vi "__Local List Menu Upload Handler.vi"(7 "FileManager Data":T1, 8 "error in (no error)":errorcluster) -> (0 "error out":errorcluster)   [LabVIEW 2011]
doc: "Handles the upload operation on the Local list."
uses:
  __File manager Data type.ctl
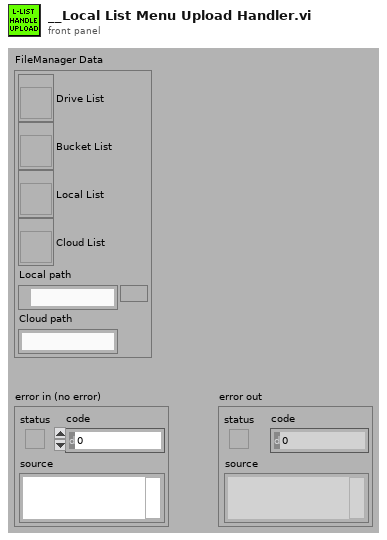
[diagram p1: front panel]
types:
  T1 = typedef "__File manager Data type.ctl" = cluster{"Drive List":refnum<vi>, "Bucket List":refnum<vi>, "Local List":refnum<vi>, "Cloud List":refnum<vi>, "Local path":path, "Cloud path":string}
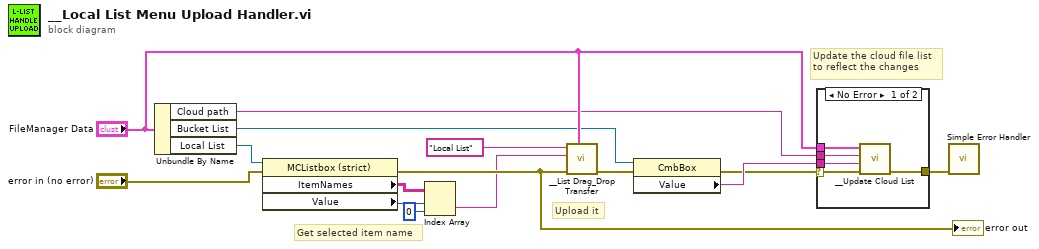
[diagram p0: block diagram]
diagram:
  # "Update the cloud file list\nto reflect the changes"
  # "Upload it"
  # "Get selected item name"
  n1 = Unbundle By Name("FileManager Data") -> ("Cloud path"=w8:string, "Bucket List"=w6:refnum<vi>, "Local List"=w15:refnum<vi>)
  n2 = property class="MCListbox (strict)"(reference=w15, error in="error in (no error)") -> (error out=w3:errorcluster, "ItemNames"=w14:string[][], "Value"=w13:i32)  [unwired: 1 out]
  "error out" <- w3
  n3 = Index Array(array=w14, index (row)=w13, index (col)=0 ("disabled index (col)")) -> (element=w1:string)
  n4 = call "__List Drag_Drop Transfer.vi"("FileManager Data"="FileManager Data", "error in (no error)"=w3, "Source Object"=w1, "Source"="Local List" ("Source Object")) -> ("error out"=w7:errorcluster)  [unwired: 7 in]
  n5 = property class="CmbBox"(reference=w6, error in=w7) -> (error out=w4:errorcluster, "Value"=w5:string)  [unwired: 1 out]
  n6 = case shown="No Error" w4 {
    selector: w4 -> [w20 w21]
    tunnel: "FileManager Data" -> [w18 _]
    tunnel: [w19 w21] -> w10
    tunnel: w8 -> [w17 _]
    tunnel: w5 -> [w16 _]
    frame No Error {
      n7 = call "__Update Cloud List.vi"("error in (no error)"=w20, "Bucket"=w16, "Path to list"=w17, "FileManager Ctl Refs in"=w18) -> ("error out"=w19:errorcluster)  [unwired: 6 in, 1 out]
    }
    frame Error {
    }
  }
  n8 = call <vilib>:"Simple Error Handler.vi"("error in (no error)"=w10) -> ()  [unwired: 4 in, 5 out]
